vi "InitCommon.vi"(8 "error in (no error)":errorcluster, 10 "AppenderConfig":T1={"id"="", "threshold"=enum."INFO", "filter"={"mode"=enum."Mirror", "levelMin"=enum."INFO", "levelMax"=enum."INFO", "tagPrefix"=""}, "queueBound"=0, "dropPolicy"=enum."DropOldest", "useUTC"=FALSE}, 11 "Appender in":refnum<class "Appender.lvclass">) -> (0 "error out":errorcluster, 3 "Appender out":refnum<class "Appender.lvclass">)   [LabVIEW 2026, in "Lumberjack.lvlib" / "Appender.lvclass"]
doc: "Populate the base appender's common private data from an AppenderConfig (id, threshold, filter, queue bound, drop policy) and zero the dropped-statement count. Called by each subclass Init after it sets its type-specific fields. Sets in-memory state only: no sink is opened (that is OpenSink on actor entry) and no config validation is performed (config is already validated upstream). Static; protected (SRS-LMBR-031)."
uses:
  Appender.lvclass
  TypeDefs/AppenderConfig.ctl
  TypeDefs/Severity.ctl
  TypeDefs/Filter.ctl
  TypeDefs/FilterMode.ctl
  TypeDefs/DropPolicy.ctl
  Appender.lvclass/Appender.ctl
  Lumberjack.lvlib
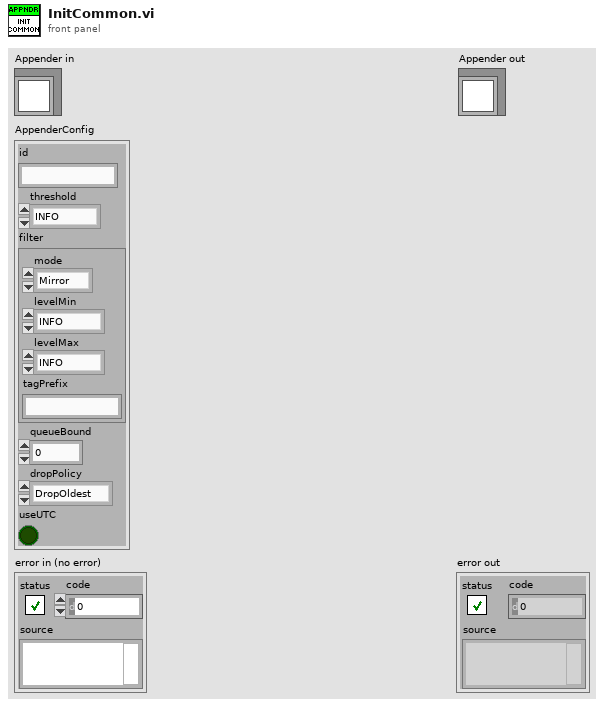
[diagram p1: front panel]
types:
  T1 = typedef "Lumberjack.lvlib/AppenderConfig.ctl" = cluster{"id":string, "threshold":T2, "filter":T3, "queueBound":i32, "dropPolicy":T5, "useUTC":bool}
  T2 = typedef "Lumberjack.lvlib/Severity.ctl" = enum16{"OFF", "FATAL", "ERROR", "WARN", "INFO", "DEBUG", "TRACE", "ALL"}
  T3 = typedef "Lumberjack.lvlib/Filter.ctl" = cluster{"mode":T4, "levelMin":T2, "levelMax":T2, "tagPrefix":string}
  T4 = typedef "Lumberjack.lvlib/FilterMode.ctl" = enum16{"Mirror", "Routed"}
  T5 = typedef "Lumberjack.lvlib/DropPolicy.ctl" = enum16{"DropOldest", "DropNewest", "LevelAware"}
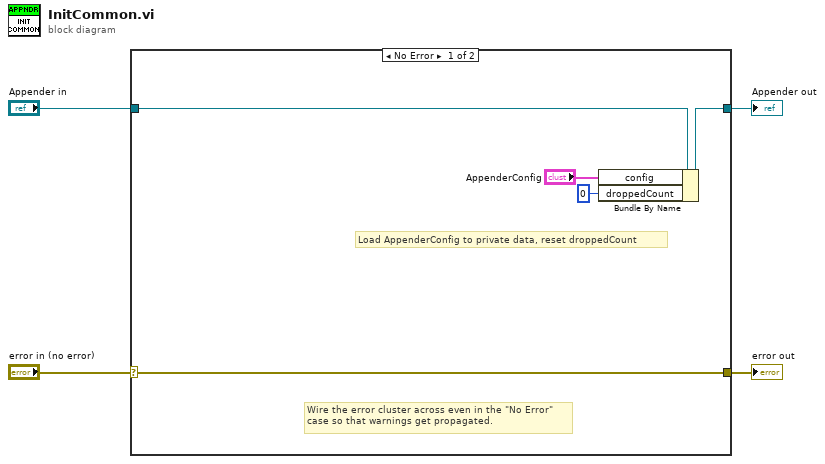
[diagram p0: block diagram]
diagram:
  n1 = case shown="No Error" "error in (no error)" {
    selector: "error in (no error)" -> [w9 w11]
    tunnel: [w9 w11] -> w3
    tunnel: [w7 w10] -> w1
    tunnel: "Appender in" -> [w8 w10]
    frame No Error {
      # "Load AppenderConfig to private data, reset droppedCount"
      # "Wire the error cluster across even in the \"No Error\"\ncase so that warnings get propagated."
      n2 = Bundle By Name(cluster=w8, "config"="AppenderConfig", "droppedCount"=u64 0) -> (w7:refnum<class "Appender.lvclass">)
    }
    frame Error {
    }
  }
  "error out" <- w3
  "Appender out" <- w1
